vi "Configure Trigger.vi"(8 "error in (no error)":errorcluster, 11 "Thermometer DAQmx Config in":refnum<class "Thermometer DAQmx Config.lvclass">) -> (0 "error out":errorcluster, 3 "Thermometer DAQmx Config out":refnum<class "Thermometer DAQmx Config.lvclass">)   [LabVIEW 2023, in "Thermometer.lvlib" / "Thermometer DAQmx.lvlib" / "Thermometer DAQmx Config.lvclass"]
uses:
  Thermometer DAQmx Config.lvclass
  Configuration Base/Configuration Base.lvclass/Configuration Base.ctl
  1ef251c9-8369-4278-8302-97e96edc9e10.vi
  <vilib>/JDP Science/JSONtext/Next JSON Value.vi
  <vilib>/JDP Science/JSONtext/String Subset.vi
  <vilib>/JDP Science/JSONtext/Parsing/Advance past next JSON Value (inlined COPY).vi
  <vilib>/JDP Science/JSONtext/Parsing/Advance past whitespace.vi
  <vilib>/JDP Science/JSONtext/Parsing/Advance past String.vi
  <vilib>/JDP Science/JSONtext/Parsing/Advance past Number.vi
  <vilib>/JDP Science/JSONtext/Parsing/Advance past Line Ending.vi
  <vilib>/JDP Science/JSONtext/Parsing/Parse Full Path or Item Name.vi
  <vilib>/JDP Science/JSONtext/Parsing/Advance past Array.vi
  <vilib>/JDP Science/JSONtext/Parsing/Advance past Object.vi
  <vilib>/JDP Science/JSONtext/support/Error Cluster From Code.vi
  <vilib>/JDP Science/JSONtext/Offset/Find Item Locations by Path.vi
  <vilib>/JDP Science/JSONtext/JSON text to Variant.vi
  <vilib>/Utility/error.llb/Error Cluster From Error Code.vi
  <vilib>/JDP Science/JSONtext/LVClass Serializer/JSONtext LVClass Serializer.lvclass
  <vilib>/ErrorRing/Error Ring.xnode
  Thermometer DAQmx Config.lvclass/Thermometer DAQmx Config.ctl
  Configuration Base/Configuration Base.lvclass
  <vilib>/JDP Science/JSONtext/JSONtext.lvlib
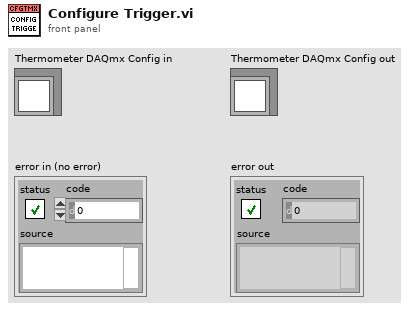
[diagram p1: front panel]
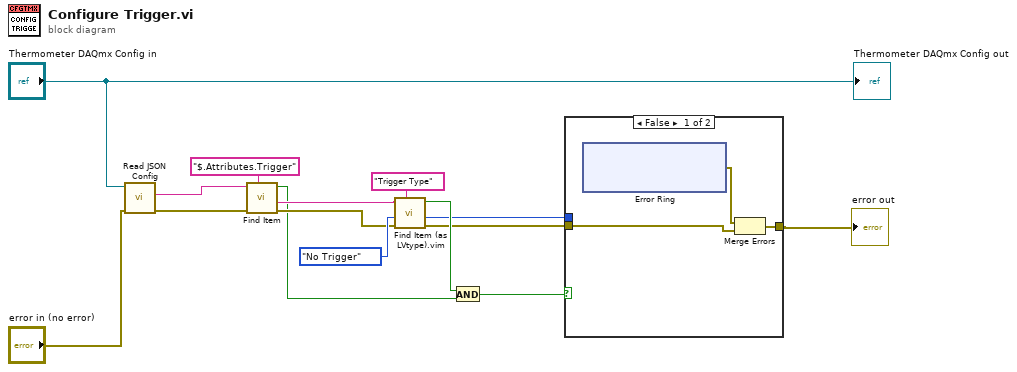
[diagram p0: block diagram]
diagram:
  n1 = call "Read JSON Config.vi"("error in"="error in (no error)", "object in"="Thermometer DAQmx Config in") -> ("error out"=w15:errorcluster, "<JSON>Config"=w14:string)  [unwired: 7 in, 1 out]
  n2 = call <vilib>:"Find Item.vi"("$Path or Item Name"="$.Attributes.Trigger", "error in (no error)"=w15, "JSON"=w14) -> ("error out"=w7:errorcluster, "<JSON>"=w10:string, "Found"=w6:bool)  [unwired: 5 in, 1 out]
  n3 = call "Find Item (as LVtype).vim"("$Path or Item Name"="Trigger Type", "error in (no error)"=w7, "Data Type and Default Value"=enum16{"No Trigger"}."No Trigger", "JSON"=w10) -> ("error out"=w3:errorcluster, "Data"=w2:enum16{"No Trigger"}, "Found"=w5:bool)  [unwired: 4 in, 1 out]
  n4 = And(x=w5, y=w6) -> (x .and. y?=w4:bool)
  n5 = case shown="False" w4 {
    tunnel: w3 -> [w17 w25]
    tunnel: w2 -> [_ w26]
    tunnel: [w16 w24] -> w1
    frame False {
      n6 = xnode "Error Ring"() -> ("error out"=w18:errorcluster)
      n7 = Merge Errors(w18, w17) -> (w16:errorcluster)
    }
    frame True {
      n8 = case shown="\"No Trigger\"" w26 {
        tunnel: w25 -> [w27 w28]
        tunnel: [w27 w28] -> w24
        frame Default {
        }
        frame "No Trigger" {
        }
      }
    }
  }
  "error out" <- w1
  "Thermometer DAQmx Config out" <- "Thermometer DAQmx Config in"
